vi "Read Values from Magna.vi"(8 "error in (no error)":errorcluster, 10 "Set Values in":T1, 11 "VISA session in":refnum<visa-resource-name>) -> (0 "error out":errorcluster, 2 "output cluster":T2, 3 "VISA session out":refnum<visa-resource-name>, 4 "Reply Expected":bool, 6 "Reply Received":bool)   [LabVIEW 2011]
uses:
  PCP interface/PCP return data types/RDd return.ctl
  PCP interface/PCP return data types/RA return Analog I.ctl
  PCP interface/PCP return data types/RP return digital IO.ctl
  Magna Configuration Values Set.ctl
  Magna PSU.lvlib
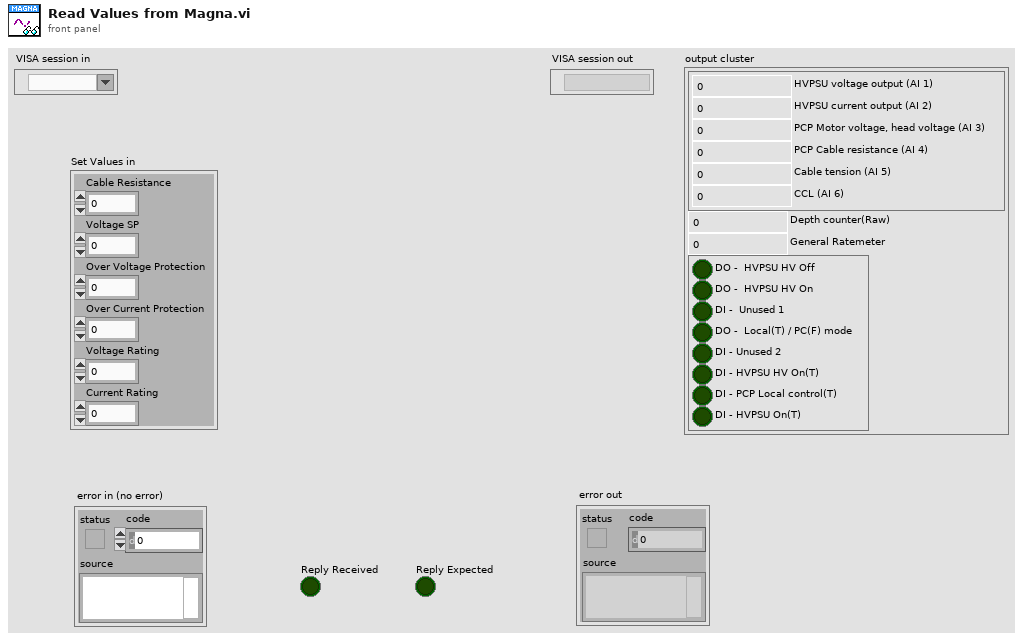
[diagram p1: front panel]
types:
  T1 = typedef "Magna Configuration Values Set.ctl" = cluster{"Cable Resistance":dbl, "Voltage SP":dbl, "Over Voltage Protection":dbl, "Over Current Protection":dbl, "Voltage Rating":dbl, "Current Rating":dbl}
  T2 = typedef "RDd return.ctl" = cluster{"AI":T3, "Depth counter(Raw)":i32, "General Ratemeter":dbl, "Digital ports":T4}
  T3 = typedef "RA return Analog I.ctl" = cluster{"HVPSU voltage output (AI 1)":dbl, "HVPSU current output (AI 2)":dbl, "PCP Motor voltage, head voltage (AI 3)":dbl, "PCP Cable resistance (AI 4)":dbl, "Cable tension (AI 5)":dbl, "CCL (AI 6)":dbl}
  T4 = typedef "RP return digital IO.ctl" = cluster{"DO -  HVPSU HV Off":bool, "DO -  HVPSU HV On":bool, "DI -  Unused 1":bool, "DO -  Local(T) / PC(F) mode":bool, "DI - Unused 2":bool, "DI - HVPSU HV On(T)":bool, "DI - PCP Local control(T)":bool, "DI - HVPSU On(T)":bool}
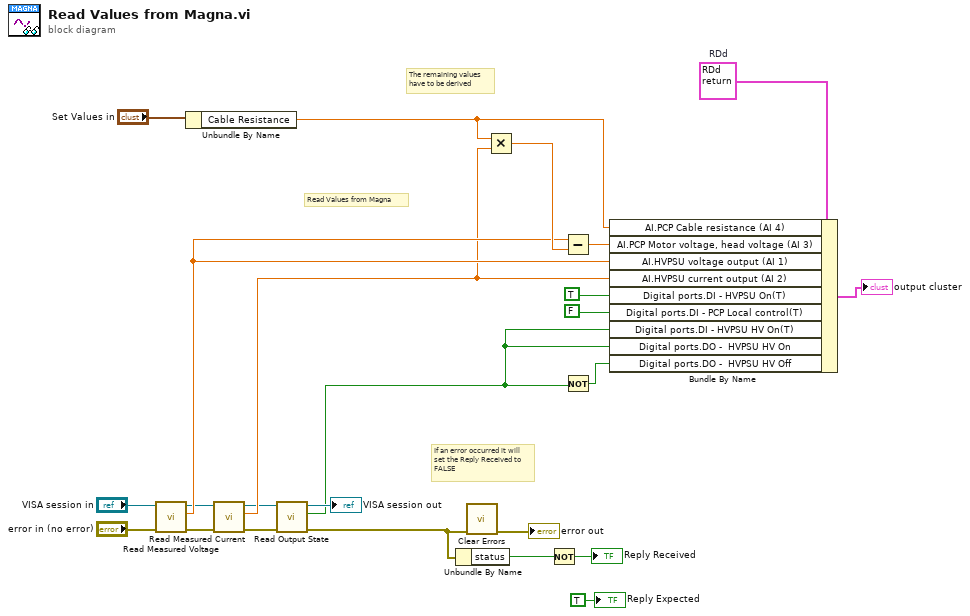
[diagram p0: block diagram]
diagram:
  w24 = T2 {"AI"={"HVPSU voltage output (AI 1)"=0.0, "HVPSU current output (AI 2)"=0.0, "PCP Motor voltage, head voltage (AI 3)"=0.0, "PCP Cable resistance (AI 4)"=0.0, "Cable tension (AI 5)"=0.0, "CCL (AI 6)"=0.0}, "Depth counter(Raw)"=0, "General Ratemeter"=0.0, "Digital ports"={"DO -  HVPSU HV Off"=FALSE, "DO -  HVPSU HV On"=FALSE, "DI -  Unused 1"=FALSE, "DO -  Local(T) / PC(F) mode"=FALSE, "DI - Unused 2"=FALSE, "DI - HVPSU HV On(T)"=FALSE, "DI - PCP Local control(T)"=FALSE, "DI - HVPSU On(T)"=FALSE}}  # RDd
  # "If an error occurred it will\nset the Reply Received to \nFALSE"
  # "The remaining values\nhave to be derived"
  # "Read Values from Magna"
  n1 = call "Read Measured Voltage.vi"("error in (no error)"="error in (no error)", "VISA session"="VISA session in") -> ("error out"=w7:errorcluster, "Voltage"=w11:dbl, "dup VISA session"=w6:refnum<visa-resource-name>)  [unwired: 7 in]
  n2 = Unbundle By Name("Set Values in") -> ("Cable Resistance"=w14:dbl)
  n3 = call "Read Measured Current.vi"("error in (no error)"=w7, "VISA session"=w6) -> ("error out"=w5:errorcluster, "Current"=w8:dbl, "dup VISA session"=w4:refnum<visa-resource-name>)  [unwired: 7 in]
  n4 = call "Read Output State.vi"("error in (no error)"=w5, "VISA session"=w4) -> ("error out"=w3:errorcluster, "Output ON"=w1:bool, "dup VISA session"=→"VISA session out":refnum<visa-resource-name>)  [unwired: 7 in]
  n5 = Unbundle By Name(w3) -> ("status"=w21:bool)
  n6 = call <vilib>:"Clear Errors.vi"("error in (no error)"=w3) -> ("error out"=→"error out":errorcluster)  [unwired: 6 in]
  n7 = Multiply(x=w14, y=w8) -> (x*y=w13:dbl)
  n8 = Not(x=w21) -> (.not. x?=→"Reply Received":bool)
  n9 = Subtract(x=w11, y=w13) -> (x-y=w12:dbl)
  n10 = Not(x=w1) -> (.not. x?=w15:bool)
  n11 = Bundle By Name(cluster=w24, "AI.PCP Cable resistance (AI 4)"=w14, "AI.PCP Motor voltage, head voltage (AI 3)"=w12, "AI.HVPSU voltage output (AI 1)"=w11, "AI.HVPSU current output (AI 2)"=w8, "Digital ports.DI - HVPSU On(T)"=TRUE, "Digital ports.DI - PCP Local control(T)"=FALSE, "Digital ports.DI - HVPSU HV On(T)"=w1, "Digital ports.DO -  HVPSU HV On"=w1, "Digital ports.DO -  HVPSU HV Off"=w15) -> (→"output cluster":T2)
  "Reply Expected" <- TRUE (".not. x? 2")
